vi "Find Max (SubVI).vi"(10 "Data 2":u8, 11 "Data 1":u8) -> (3 "Max":u8)   [LabVIEW 2015]
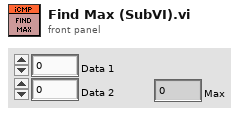
[diagram p1: front panel]
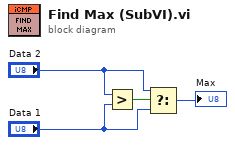
[diagram p0: block diagram]
diagram:
  n1 = Greater?(x="Data 2", y="Data 1") -> (0:w2:bool)
  n2 = Select(t="Data 2", s=w2, f="Data 1") -> (s? t:f=→"Max":u8)
